vi "Array To Matrix.vi"   [LabVIEW 2020, in "NI_Matrix.lvlib"]
doc: "Converts an array to a matrix of elements of the same type as the array elements. Wire data to the <B>Real 2D Array</B> input to determine the polymorphic instance to use or manually select the instance."
uses:
  <vilib>/Analysis/Matrix/NI_Matrix.lvlib
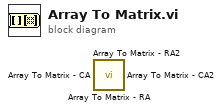
[diagram p0: block diagram]
diagram:
  n1 = call <vilib>:"Array To Matrix - RA.vi"() -> ()  [unwired: 1 in, 1 out]
  n2 = call <vilib>:"Array To Matrix - RA2.vi"() -> ()  [unwired: 1 in, 1 out]
  n3 = call <vilib>:"Array To Matrix - CA.vi"() -> ()  [unwired: 1 in, 1 out]
  n4 = call <vilib>:"Array To Matrix - CA2.vi"() -> ()  [unwired: 1 in, 1 out]
